vi "UTILITY Queue.vi"(6 "timeout in ms (-1)":i32, 7 "Status":T1, 8 "error in (no error)":errorcluster, 10 "Set Status":bool, 11 "name (unnamed)":string) -> (0 "error out":errorcluster, 2 "timed out?":bool, 3 "latest READ notification":bool)   [LabVIEW 2014]
uses:
  Type Definitions/UTILITY Notifier.ctl
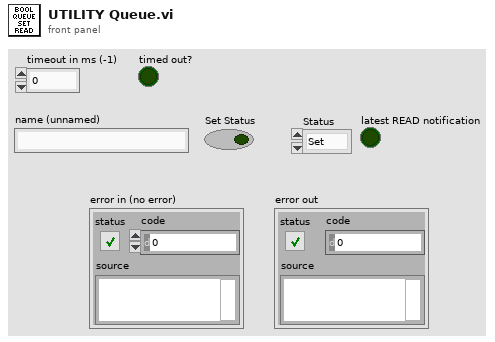
[diagram p1: front panel]
types:
  T1 = typedef "UTILITY Notifier.ctl" = enum16{"Set", "Read", "Release Ref"}
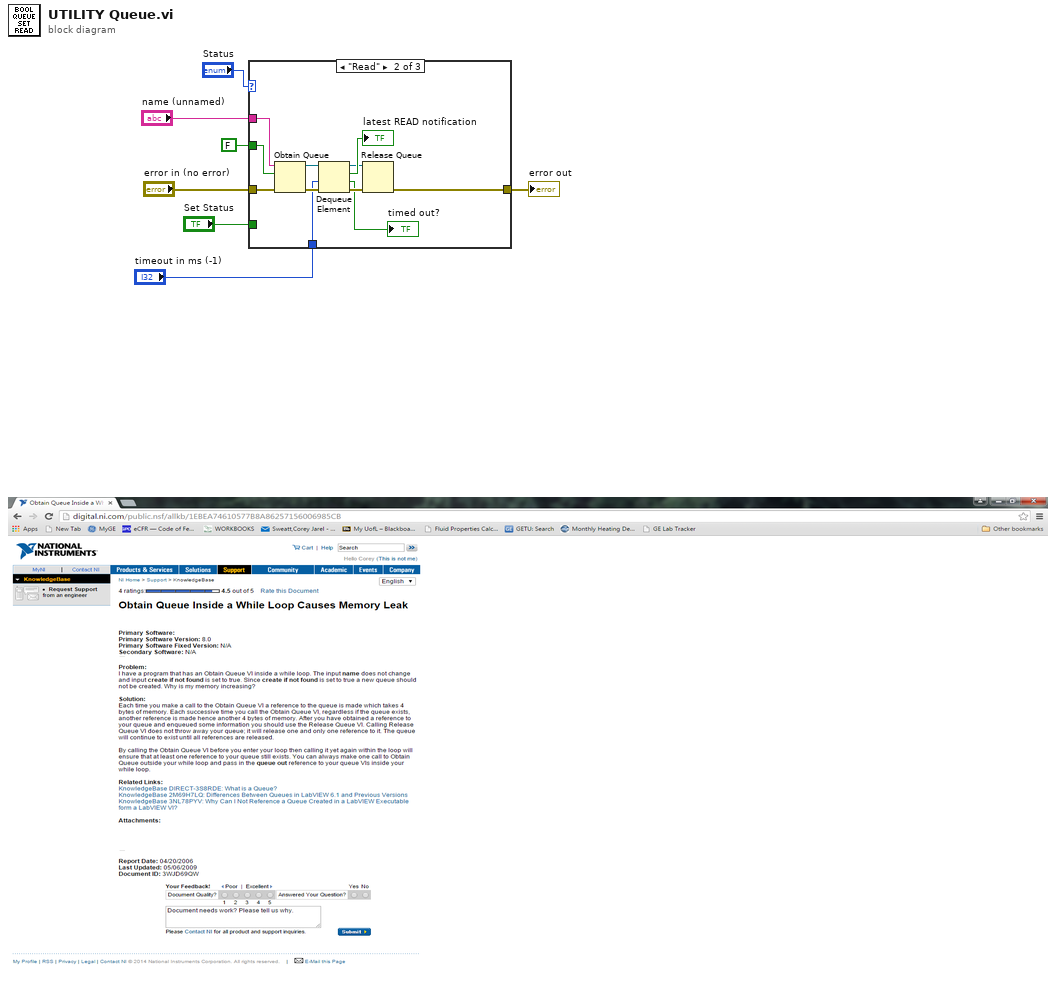
[diagram p0: block diagram]
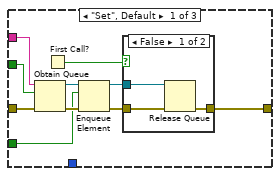
[diagram p2: hidden frame]
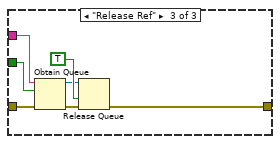
[diagram p4: hidden frame]
diagram:
  n1 = case shown="\"Read\"" "Status" {
    tunnel: [w17 w25 w37] -> w7
    tunnel: "error in (no error)" -> [w12 w32 w39]
    tunnel: "name (unnamed)" -> [w14 w31 w34]
    tunnel: "Set Status" -> [w8 _ _]
    tunnel: FALSE ("Aisle 1 Update") -> [w13 w30 w33]
    tunnel: "timeout in ms (-1)" -> [_ w23 _]
    frame "Set", Default {
      n2 = Obtain Queue(name (unnamed)=w14, element data type=w13, error in (no error)=w12) -> (queue out=w15:refnum<queue>, error out=w11:errorcluster)  [unwired: 2 in, 1 out]
      n3 = First Call?() -> (First Call?: T/F=w16:bool)
      n4 = Enqueue Element(queue=w15, element=w8, error in (no error)=w11) -> (queue out=w9:refnum<queue>, error out=w10:errorcluster)  [unwired: 1 in, 1 out]
      n5 = case shown="False" w16 {
        tunnel: w10 -> [w20 w21]
        tunnel: [w19 w21] -> w17
        tunnel: w9 -> [w18 _]
        frame False {
          n6 = Release Queue(queue=w18, error in (no error)=w20) -> (error out=w19:errorcluster)  [unwired: 1 in, 2 out]
        }
        frame True {
        }
      }
    }
    frame "Read" {
      n7 = Obtain Queue(name (unnamed)=w31, element data type=w30, error in (no error)=w32) -> (queue out=w28:refnum<queue>, error out=w29:errorcluster)  [unwired: 2 in, 1 out]
      n8 = Dequeue Element(queue=w28, timeout in ms (-1)=w23, error in (no error)=w29) -> (queue out=w24:refnum<queue>, element=→"latest READ notification":bool, timed out?=→"timed out?":bool, error out=w26:errorcluster)
      n9 = Release Queue(queue=w24, error in (no error)=w26) -> (error out=w25:errorcluster)  [unwired: 1 in, 2 out]
    }
    frame "Release Ref" {
      n10 = Obtain Queue(name (unnamed)=w34, element data type=w33, error in (no error)=w39) -> (queue out=w35:refnum<queue>, error out=w38:errorcluster)  [unwired: 2 in, 1 out]
      n11 = Release Queue(queue=w35, force destroy? (F)=TRUE, error in (no error)=w38) -> (error out=w37:errorcluster)  [unwired: 2 out]
    }
  }
  "error out" <- w7
